vi "Add Block Diagram Content.vi"(8 "error in (no error)":errorcluster, 9 "Term Refnum":refnum<vi>, 10 "ModuleLoop":T1, 11 "EST Digital Event in":refnum<class "Digital Event.lvclass">) -> (0 "error out":errorcluster, 3 "EST Digital Event out":refnum<class "Digital Event.lvclass">)   [LabVIEW 2015, in "Digital Event.lvclass"]
uses:
  Digital Event.lvclass
  Loop/Block Diagram/Module.Refs.ctl
  <vilib>/Utility/miscctls.llb/LVPointTypeDef.ctl
  Loop/Structures/Structures.lvclass
  Loop/Block Diagram/Block Diagram.lvclass
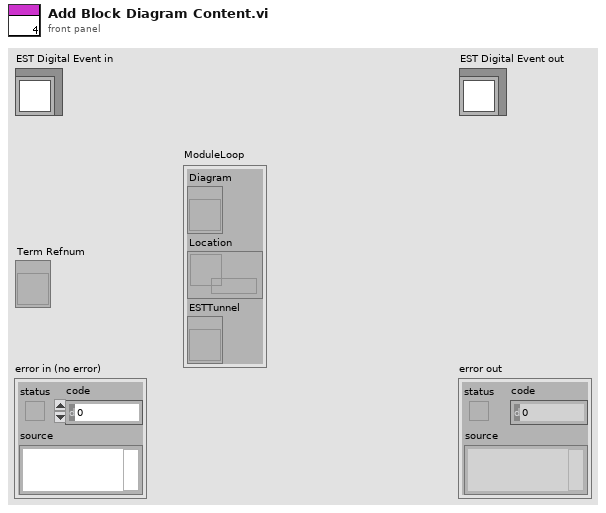
[diagram p1: front panel]
types:
  T1 = typedef "Block Diagram.lvclass/Module.Refs.ctl" = cluster{"Diagram":refnum<vi>, "Location":refnum<data-value>, "ESTTunnel":refnum<vi>}
  T2 = typedef "LVPointTypeDef.ctl" = cluster{"Horizontal":i16, "Vertical":i16}
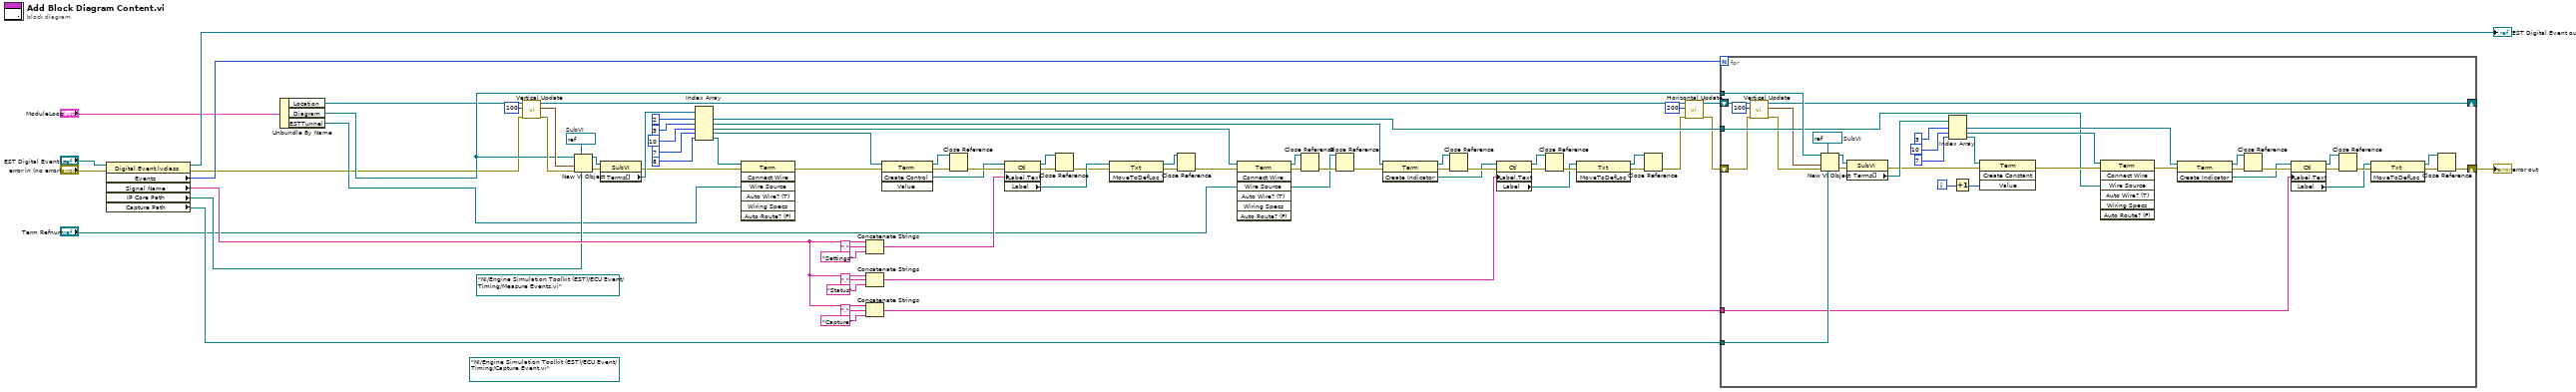
[diagram p0: block diagram]
diagram:
  (unwired) path "NI/Engine Simulation Toolkit (EST)/ECU Event/Timing/Measure Events.vi" ("path")
  (unwired) path "NI/Engine Simulation Toolkit (EST)/ECU Event/Timing/Capture Event.vi" ("path")
  w51 = refnum<vi> refnum  # SubVI
  n1 = property class="Digital Event.lvclass"(reference="EST Digital Event in", error in="error in (no error)") -> (reference out=→"EST Digital Event out":refnum<class "Digital Event.lvclass">, error out=w1:errorcluster, "Events"=w20:u32, "Signal Name"=w19:string, "IP Core Path"=w18:path, "Capture Path"=w17:path)
  n2 = Unbundle By Name("ModuleLoop") -> ("Location"=w2:refnum<data-value>, "Diagram"=w3:refnum<vi>, "ESTTunnel"=w4:refnum<vi>)
  n3 = call "Vertical Update.vi"("error in (no error)"=w1, "Vertical Change"=i16 100, "Location"=w2) -> ("error out"=w14:errorcluster, "location out"=w13:T2, "Location"=w12:refnum<data-value>)  [unwired: 6 in]
  n4 = New VI Object(vi object class=w51, owner refnum=w3, position/next to=w13, 6:w18, 8:w14) -> (object refnum=w53:refnum<vi>, 0:w54:errorcluster)  [unwired: 3 in]
  n5 = property class="SubVI"(reference=w53, error in=w54) -> (error out=w24:errorcluster, "Terms[]"=w52:refnum<vi>[])  [unwired: 1 out]
  n6 = Index Array(array=w52, index #1=2 ("index"), index #2=3 ("index"), index #3=10 ("index"), index #4=7 ("index"), index #5=8 ("index")) -> (element #1=w30:refnum<vi>, element #2=w32:refnum<vi>, element #3=w33:refnum<vi>, element #4=w34:refnum<vi>, element #5=w25:refnum<vi>)
  n7 = invoke class="Term" method="Connect Wire"(reference=w25, error in=w24, "Wire Source"=w4) -> (error out=w23:errorcluster)  [unwired: 4 in, 6 out]
  n8 = Concatenate Strings(w19, "." ("string"), "Settings" ("string")) -> (w55:string)
  n9 = Concatenate Strings(w19, "." ("string"), "Status" ("string")) -> (w31:string)
  n10 = Concatenate Strings(w19, "." ("string"), "Capture" ("string")) -> (w27:string)
  n11 = invoke class="Term" method="Create Control"(reference=w34, error in=w23) -> (reference out=w62:refnum<vi>, error out=w61:errorcluster, "Create Control"=w50:refnum<vi>)  [unwired: 2 in, 1 out]
  n12 = Close Reference(reference=w62, error in (no error)=w61) -> (error out=w63:errorcluster)
  n13 = property class="Ctl"(reference=w50, error in=w63, "Label.Text"=w55) -> (reference out=w49:refnum<vi>, error out=w47:errorcluster, "Label"=w48:refnum<vi>)
  n14 = Close Reference(reference=w49, error in (no error)=w47) -> (error out=w46:errorcluster)
  n15 = invoke class="Txt" method="MoveToDefLoc"(reference=w48, error in=w46) -> (reference out=w44:refnum<vi>, error out=w45:errorcluster)  [unwired: 1 in, 1 out]
  n16 = Close Reference(reference=w44, error in (no error)=w45) -> (error out=w43:errorcluster)
  n17 = invoke class="Term" method="Connect Wire"(reference=w33, error in=w43, "Wire Source"="Term Refnum") -> (reference out=w65:refnum<vi>, error out=w64:errorcluster)  [unwired: 4 in, 5 out]
  n18 = Close Reference(reference=w65, error in (no error)=w64) -> (error out=w66:errorcluster)
  n19 = Close Reference(reference="Term Refnum", error in (no error)=w66) -> (error out=w67:errorcluster)
  n20 = invoke class="Term" method="Create Indicator"(reference=w32, error in=w67) -> (reference out=w70:refnum<vi>, error out=w71:errorcluster, "Create Indicator"=w58:refnum<vi>)  [unwired: 1 in]
  n21 = Close Reference(reference=w70, error in (no error)=w71) -> (error out=w72:errorcluster)
  n22 = property class="Ctl"(reference=w58, error in=w72, "Label.Text"=w31) -> (reference out=w68:refnum<vi>, error out=w69:errorcluster, "Label"=w40:refnum<vi>)
  n23 = Close Reference(reference=w68, error in (no error)=w69) -> (error out=w41:errorcluster)
  n24 = invoke class="Txt" method="MoveToDefLoc"(reference=w40, error in=w41) -> (reference out=w39:refnum<vi>, error out=w42:errorcluster)  [unwired: 1 in, 1 out]
  n25 = Close Reference(reference=w39, error in (no error)=w42) -> (error out=w9:errorcluster)
  n26 = call "Horizontal Update.vi"("error in (no error)"=w9, "Horizontal Change"=i16 200 ("Vertical Change"), "Location"=w12) -> ("error out"=w8:errorcluster, "Location"=w10:refnum<data-value>)  [unwired: 6 in, 1 out]
  n27 = for {
    N: w20 -> [_]
    shift-right: [w88] -> w7
    shift-left: w8 -> [w74]
    tunnel: w3 -> [w105]
    tunnel: w17 -> [w104]
    tunnel: w27 -> [w87]
    tunnel: w30 -> [w79]
    shift-right: [w77] -> _
    shift-left: w10 -> [w75]
    i -> [w84]
    w106 = refnum<vi> refnum  # SubVI
    n28 = call "Vertical Update.vi"("error in (no error)"=w74, "Vertical Change"=i16 100, "Location"=w75) -> ("error out"=w73:errorcluster, "location out"=w76:T2, "Location"=w77:refnum<data-value>)  [unwired: 6 in]
    n29 = New VI Object(vi object class=w106, owner refnum=w105, position/next to=w76, 6:w104, 8:w73) -> (object refnum=w107:refnum<vi>, 0:w108:errorcluster)  [unwired: 3 in]
    n30 = property class="SubVI"(reference=w107, error in=w108) -> (error out=w85:errorcluster, "Terms[]"=w103:refnum<vi>[])  [unwired: 1 out]
    n31 = Index Array(array=w103, index #1=3 ("index"), index #2=10 ("index"), index #3=7 ("index")) -> (element #1=w89:refnum<vi>, element #2=w82:refnum<vi>, element #3=w86:refnum<vi>)
    n32 = Increment(x=w84) -> (x+1=w83:i32)
    n33 = invoke class="Term" method="Create Constant"(reference=w86, error in=w85, "Value"=w83) -> (error out=w81:errorcluster)  [unwired: 1 in, 3 out]
    n34 = invoke class="Term" method="Connect Wire"(reference=w82, error in=w81, "Wire Source"=w79) -> (error out=w80:errorcluster)  [unwired: 4 in, 6 out]
    n35 = invoke class="Term" method="Create Indicator"(reference=w89, error in=w80) -> (reference out=w97:refnum<vi>, error out=w98:errorcluster, "Create Indicator"=w94:refnum<vi>)  [unwired: 1 in]
    n36 = Close Reference(reference=w97, error in (no error)=w98) -> (error out=w99:errorcluster)
    n37 = property class="Ctl"(reference=w94, error in=w99, "Label.Text"=w87) -> (reference out=w95:refnum<vi>, error out=w96:errorcluster, "Label"=w91:refnum<vi>)
    n38 = Close Reference(reference=w95, error in (no error)=w96) -> (error out=w92:errorcluster)
    n39 = invoke class="Txt" method="MoveToDefLoc"(reference=w91, error in=w92) -> (reference out=w90:refnum<vi>, error out=w93:errorcluster)  [unwired: 1 in, 1 out]
    n40 = Close Reference(reference=w90, error in (no error)=w93) -> (error out=w88:errorcluster)
  }
  "error out" <- w7
